vi "Generate Report.vi"(7 "Data_In":T1={"Input Data 1D"=[], "Channel Settings"={"Supply Voltage [Vdc]"=0.0, "Max Supply Current [Idc]"=0.0, "Settling Delay"=0.0, "Temp Criteria"=0.0, "Voltage Steps [Vrms]"=[0.0, 0.25, 0.5, 1.0, 1.95, 3.0, 3.9, 5.5], "User Notes"="", "Config Wave File Path"=path "C:/ASD Power Point Beta 32J/Waveforms/150HzSine5Second.wav", "Config Voltage [Vrms]"=0.0, "Channel Configuration List"={"Channel Configuration Cluster"={"Input"=enum."---", "Enable"=FALSE, "User Notes"="", "Voltage Range"=0.0, "Current Range"=2.5}, "Channel Configuration Cluster 2"={"Input"=enum."---", "Enable"=FALSE, "User Notes"="", "Voltage Range"=0.0, "Current Range"=2.5}, "Channel Configuration Cluster 3"={"Input"=enum."---", "Enable"=FALSE, "User Notes"="", "Voltage Range"=0.0, "Current Range"=2.5}, "Channel Configuration Cluster 4"={"Input"=enum."---", "Enable"=FALSE, "User Notes"="", "Voltage Range"=0.0, "Current Range"=2.5}, "Channel Configuration Cluster 5"={"Input"=enum."---", "Enable"=FALSE, "User Notes"="", "Voltage Range"=0.0, "Current Range"=2.5}, "Channel Configuration Cluster 6"={"Input"=enum."---", "Enable"=FALSE, "User Notes"="", "Voltage Range"=0.0, "Current Range"=2.5}, "Channel Configuration Cluster 7"={"Input"=enum."---", "Enable"=FALSE, "User Notes"="", "Voltage Range"=0.0, "Current Range"=2.5}, "Channel Configuration Cluster 8"={"Input"=enum."---", "Enable"=FALSE, "User Notes"="", "Voltage Range"=0.0, "Current Range"=2.5}, "Channel Configuration Cluster 9"={"Input"=enum."---", "Enable"=FALSE, "User Notes"="", "Voltage Range"=0.0, "Current Range"=2.5}, "Channel Configuration Cluster 10"={"Input"=enum."---", "Enable"=FALSE, "User Notes"="", "Voltage Range"=0.0, "Current Range"=2.5}, "Channel Configuration Cluster 11"={"Input"=enum."---", "Enable"=FALSE, "User Notes"="", "Voltage Range"=0.0, "Current Range"=2.5}, "Channel Configuration Cluster 12"={"Input"=enum."---", "Enable"=FALSE, "User Notes"="", "Voltage Range"=0.0, "Current Range"=2.5}, "Channel Configuration Cluster 13"={"Input"=enum."---", "Enable"=FALSE, "User Notes"="", "Voltage Range"=0.0, "Current Range"=2.5}, "Channel Configuration Cluster 14"={"Input"=enum."---", "Enable"=FALSE, "User Notes"="", "Voltage Range"=0.0, "Current Range"=2.5}, "Channel Configuration Cluster 15"={"Input"=enum."---", "Enable"=FALSE, "User Notes"="", "Voltage Range"=0.0, "Current Range"=2.5}, "Channel Configuration Cluster 16"={"Input"=enum."---", "Enable"=FALSE, "User Notes"="", "Voltage Range"=0.0, "Current Range"=2.5}, "Channel Configuration Cluster 17"={"Input"=enum."---", "Enable"=FALSE, "User Notes"="", "Voltage Range"=0.0, "Current Range"=2.5}}, "User Gains"={"Gain 1"=0.0, "Gain 2"=0.0, "Gain 3"=0.0, "Gain 4"=0.0, "Gain 5"=0.0, "Gain 6"=0.0}, "Gains"={"Gain 1"=0.0, "Gain 2"=0.0, "Gain 3"=0.0, "Gain 4"=0.0, "Gain 5"=0.0, "Gain 6"=0.0}, "Gain Array"={"Gain 1"=0.0, "Gain 2"=0.0, "Gain 3"=0.0, "Gain 4"=0.0, "Gain 5"=0.0, "Gain 6"=0.0, "Gain 7"=0.0, "Gain 8"=0.0, "Gain 9"=0.0, "Gain 10"=0.0, "Gain 11"=0.0, "Gain 12"=0.0, "Gain 13"=0.0, "Gain 14"=0.0, "Gain 15"=0.0, "Gain 16"=0.0, "Gain 17"=0.0}, "Wave File Path 1"=path "", "Wave File Path 2"=path "", "Wave File Path 3"=path "", "Wave File Path 4"=path "", "Range"=FALSE, "CF"=FALSE}, "Select Data"={"Vrms Data"=FALSE, "Vpkpk Data"=FALSE, "Irms Data"=FALSE, "Power Data"=FALSE, "Ipkpk Data"=FALSE, "Temp Data"=FALSE}, "Detailed Report ?"=FALSE, "Path Settings:"={"Template Path "=path "E:/L&T Projects/Bose ASD/Excel Template/ASD Template.xltx", "Report Path"=path "E:/L&T Projects/Bose ASD/excel Reports", "JPEG1 Path "=path "C:/Users/Public/Pictures/Sample Pictures/Hydrangeas.jpg", "JPEG2 Path"=path "C:/Users/Public/Pictures/Sample Pictures/Lighthouse.jpg"}, "Vrms_Sheet"=[], "Irms_Sheet"=[], "Power_Sheet"=[], "Vpk_Sheet"=[], "Ipk_Sheet"=[], "Vrms_Avg"=[], "Irms_Avg"=[], "Power_Avg"=[], "Vpk_Avg"=[], "Ipk_Avg"=[], "Report_Ref"=refnum, "User Name"="", "Temp_Sheet"=[]} {"Channel Settings"."Gain Array"."Gain 17" format="%.2f"; "Channel Settings"."Gain Array"."Gain 16" format="%.2f"; "Channel Settings"."Gain Array"."Gain 15" format="%.2f"; "Channel Settings"."Gain Array"."Gain 14" format="%.2f"; "Channel Settings"."Gain Array"."Gain 13" format="%.2f"; "Channel Settings"."Gain Array"."Gain 12" format="%.2f"; "Channel Settings"."Gain Array"."Gain 11" format="%.2f"; "Channel Settings"."Gain Array"."Gain 10" format="%.2f"; "Channel Settings"."Gain Array"."Gain 9" format="%.2f"; "Channel Settings"."Gain Array"."Gain 8" format="%.2f"; "Channel Settings"."Gain Array"."Gain 7" format="%.2f"; "Channel Settings"."Gain Array"."Gain 6" format="%.2f"; "Channel Settings"."Gain Array"."Gain 5" format="%.2f"; "Channel Settings"."Gain Array"."Gain 4" format="%.2f"; "Channel Settings"."Gain Array"."Gain 3" format="%.2f"; "Channel Settings"."Gain Array"."Gain 2" format="%.2f"; "Channel Settings"."Gain Array"."Gain 1" format="%.2f"; "Channel Settings"."Gains"."Gain 6" format="%.2f"; "Channel Settings"."Gains"."Gain 5" format="%.2f"; "Channel Settings"."Gains"."Gain 4" format="%.2f"; "Channel Settings"."Gains"."Gain 3" format="%.2f"; "Channel Settings"."Gains"."Gain 2" format="%.2f"; "Channel Settings"."Gains"."Gain 1" format="%.2f"; "Channel Settings"."User Gains"."Gain 6" format="%.2f"; "Channel Settings"."User Gains"."Gain 5" format="%.2f"; "Channel Settings"."User Gains"."Gain 4" format="%.2f"; "Channel Settings"."User Gains"."Gain 3" format="%.2f"; "Channel Settings"."User Gains"."Gain 2" format="%.2f"; "Channel Settings"."User Gains"."Gain 1" format="%.2f"; "Channel Settings"."Channel Configuration List"."Channel Configuration Cluster 17"."Current Range" items=["1 <500m>"=0.5, "2 <1>"=1.0, "5 <2.5>"=2.5, "10 <5>"=5.0, "20 <10>"=10.0, "50 <25>"=25.0]; "Channel Settings"."Channel Configuration List"."Channel Configuration Cluster 17"."Voltage Range" items=["1.5 <0.75>"=0.75, "3 <1.5>"=1.5, "6 <3>"=3.0, "10 <5>"=5.0, "15 <7.5>"=7.5, "30 <15>"=15.0, "60 <30>"=30.0, "100 <50>"=50.0, "150 <75>"=75.0, "300 <150>"=150.0, "600 <300>"=300.0, "1000 <500>"=500.0]; "Channel Settings"."Channel Configuration List"."Channel Configuration Cluster 16"."Current Range" items=["1 <500m>"=0.5, "2 <1>"=1.0, "5 <2.5>"=2.5, "10 <5>"=5.0, "20 <10>"=10.0, "50 <25>"=25.0]; "Channel Settings"."Channel Configuration List"."Channel Configuration Cluster 16"."Voltage Range" items=["1.5 <0.75>"=0.75, "3 <1.5>"=1.5, "6 <3>"=3.0, "10 <5>"=5.0, "15 <7.5>"=7.5, "30 <15>"=15.0, "60 <30>"=30.0, "100 <50>"=50.0, "150 <75>"=75.0, "300 <150>"=150.0, "600 <300>"=300.0, "1000 <500>"=500.0]; "Channel Settings"."Channel Configuration List"."Channel Configuration Cluster 15"."Current Range" items=["1 <500m>"=0.5, "2 <1>"=1.0, "5 <2.5>"=2.5, "10 <5>"=5.0, "20 <10>"=10.0, "50 <25>"=25.0]; "Channel Settings"."Channel Configuration List"."Channel Configuration Cluster 15"."Voltage Range" items=["1.5 <0.75>"=0.75, "3 <1.5>"=1.5, "6 <3>"=3.0, "10 <5>"=5.0, "15 <7.5>"=7.5, "30 <15>"=15.0, "60 <30>"=30.0, "100 <50>"=50.0, "150 <75>"=75.0, "300 <150>"=150.0, "600 <300>"=300.0, "1000 <500>"=500.0]; "Channel Settings"."Channel Configuration List"."Channel Configuration Cluster 14"."Current Range" items=["1 <500m>"=0.5, "2 <1>"=1.0, "5 <2.5>"=2.5, "10 <5>"=5.0, "20 <10>"=10.0, "50 <25>"=25.0]; "Channel Settings"."Channel Configuration List"."Channel Configuration Cluster 14"."Voltage Range" items=["1.5 <0.75>"=0.75, "3 <1.5>"=1.5, "6 <3>"=3.0, "10 <5>"=5.0, "15 <7.5>"=7.5, "30 <15>"=15.0, "60 <30>"=30.0, "100 <50>"=50.0, "150 <75>"=75.0, "300 <150>"=150.0, "600 <300>"=300.0, "1000 <500>"=500.0]; "Channel Settings"."Channel Configuration List"."Channel Configuration Cluster 13"."Current Range" items=["1 <500m>"=0.5, "2 <1>"=1.0, "5 <2.5>"=2.5, "10 <5>"=5.0, "20 <10>"=10.0, "50 <25>"=25.0]; "Channel Settings"."Channel Configuration List"."Channel Configuration Cluster 13"."Voltage Range" items=["1.5 <0.75>"=0.75, "3 <1.5>"=1.5, "6 <3>"=3.0, "10 <5>"=5.0, "15 <7.5>"=7.5, "30 <15>"=15.0, "60 <30>"=30.0, "100 <50>"=50.0, "150 <75>"=75.0, "300 <150>"=150.0, "600 <300>"=300.0, "1000 <500>"=500.0]; "Channel Settings"."Channel Configuration List"."Channel Configuration Cluster 12"."Current Range" items=["1 <500m>"=0.5, "2 <1>"=1.0, "5 <2.5>"=2.5, "10 <5>"=5.0, "20 <10>"=10.0, "50 <25>"=25.0]; "Channel Settings"."Channel Configuration List"."Channel Configuration Cluster 12"."Voltage Range" items=["1.5 <0.75>"=0.75, "3 <1.5>"=1.5, "6 <3>"=3.0, "10 <5>"=5.0, "15 <7.5>"=7.5, "30 <15>"=15.0, "60 <30>"=30.0, "100 <50>"=50.0, "150 <75>"=75.0, "300 <150>"=150.0, "600 <300>"=300.0, "1000 <500>"=500.0]; "Channel Settings"."Channel Configuration List"."Channel Configuration Cluster 11"."Current Range" items=["1 <500m>"=0.5, "2 <1>"=1.0, "5 <2.5>"=2.5, "10 <5>"=5.0, "20 <10>"=10.0, "50 <25>"=25.0]; "Channel Settings"."Channel Configuration List"."Channel Configuration Cluster 11"."Voltage Range" items=["1.5 <0.75>"=0.75, "3 <1.5>"=1.5, "6 <3>"=3.0, "10 <5>"=5.0, "15 <7.5>"=7.5, "30 <15>"=15.0, "60 <30>"=30.0, "100 <50>"=50.0, "150 <75>"=75.0, "300 <150>"=150.0, "600 <300>"=300.0, "1000 <500>"=500.0]; "Channel Settings"."Channel Configuration List"."Channel Configuration Cluster 10"."Current Range" items=["1 <500m>"=0.5, "2 <1>"=1.0, "5 <2.5>"=2.5, "10 <5>"=5.0, "20 <10>"=10.0, "50 <25>"=25.0]; "Channel Settings"."Channel Configuration List"."Channel Configuration Cluster 10"."Voltage Range" items=["1.5 <0.75>"=0.75, "3 <1.5>"=1.5, "6 <3>"=3.0, "10 <5>"=5.0, "15 <7.5>"=7.5, "30 <15>"=15.0, "60 <30>"=30.0, "100 <50>"=50.0, "150 <75>"=75.0, "300 <150>"=150.0, "600 <300>"=300.0, "1000 <500>"=500.0]; "Channel Settings"."Channel Configuration List"."Channel Configuration Cluster 9"."Voltage Range" items=["1.5 <0.75>"=0.75, "3 <1.5>"=1.5, "6 <3>"=3.0, "10 <5>"=5.0, "15 <7.5>"=7.5, "30 <15>"=15.0, "60 <30>"=30.0, "100 <50>"=50.0, "150 <75>"=75.0, "300 <150>"=150.0, "600 <300>"=300.0, "1000 <500>"=500.0]; "Channel Settings"."Channel Configuration List"."Channel Configuration Cluster 9"."Current Range" items=["10m <5m>"=0.005, "20m <10m>"=0.01, "50m <25m>"=0.025, "100m <50m>"=0.05, "200m <100m>"=0.1, "500m <250m>"=0.25, "1 <500m>"=0.5, "2 <1>"=1.0, "5 <2.5>"=2.5]; "Channel Settings"."Channel Configuration List"."Channel Configuration Cluster 8"."Voltage Range" items=["1.5 <0.75>"=0.75, "3 <1.5>"=1.5, "6 <3>"=3.0, "10 <5>"=5.0, "15 <7.5>"=7.5, "30 <15>"=15.0, "60 <30>"=30.0, "100 <50>"=50.0, "150 <75>"=75.0, "300 <150>"=150.0, "600 <300>"=300.0, "1000 <500>"=500.0]; "Channel Settings"."Channel Configuration List"."Channel Configuration Cluster 8"."Current Range" items=["10m <5m>"=0.005, "20m <10m>"=0.01, "50m <25m>"=0.025, "100m <50m>"=0.05, "200m <100m>"=0.1, "500m <250m>"=0.25, "1 <500m>"=0.5, "2 <1>"=1.0, "5 <2.5>"=2.5]; "Channel Settings"."Channel Configuration List"."Channel Configuration Cluster 7"."Voltage Range" items=["1.5 <0.75>"=0.75, "3 <1.5>"=1.5, "6 <3>"=3.0, "10 <5>"=5.0, "15 <7.5>"=7.5, "30 <15>"=15.0, "60 <30>"=30.0, "100 <50>"=50.0, "150 <75>"=75.0, "300 <150>"=150.0, "600 <300>"=300.0, "1000 <500>"=500.0]; "Channel Settings"."Channel Configuration List"."Channel Configuration Cluster 7"."Current Range" items=["10m <5m>"=0.005, "20m <10m>"=0.01, "50m <25m>"=0.025, "100m <50m>"=0.05, "200m <100m>"=0.1, "500m <250m>"=0.25, "1 <500m>"=0.5, "2 <1>"=1.0, "5 <2.5>"=2.5]; "Channel Settings"."Channel Configuration List"."Channel Configuration Cluster 6"."Voltage Range" items=["1.5 <0.75>"=0.75, "3 <1.5>"=1.5, "6 <3>"=3.0, "10 <5>"=5.0, "15 <7.5>"=7.5, "30 <15>"=15.0, "60 <30>"=30.0, "100 <50>"=50.0, "150 <75>"=75.0, "300 <150>"=150.0, "600 <300>"=300.0, "1000 <500>"=500.0]; "Channel Settings"."Channel Configuration List"."Channel Configuration Cluster 6"."Current Range" items=["10m <5m>"=0.005, "20m <10m>"=0.01, "50m <25m>"=0.025, "100m <50m>"=0.05, "200m <100m>"=0.1, "500m <250m>"=0.25, "1 <500m>"=0.5, "2 <1>"=1.0, "5 <2.5>"=2.5]; "Channel Settings"."Channel Configuration List"."Channel Configuration Cluster 5"."Voltage Range" items=["1.5 <0.75>"=0.75, "3 <1.5>"=1.5, "6 <3>"=3.0, "10 <5>"=5.0, "15 <7.5>"=7.5, "30 <15>"=15.0, "60 <30>"=30.0, "100 <50>"=50.0, "150 <75>"=75.0, "300 <150>"=150.0, "600 <300>"=300.0, "1000 <500>"=500.0]; "Channel Settings"."Channel Configuration List"."Channel Configuration Cluster 5"."Current Range" items=["10m <5m>"=0.005, "20m <10m>"=0.01, "50m <25m>"=0.025, "100m <50m>"=0.05, "200m <100m>"=0.1, "500m <250m>"=0.25, "1 <500m>"=0.5, "2 <1>"=1.0, "5 <2.5>"=2.5]; "Channel Settings"."Channel Configuration List"."Channel Configuration Cluster 4"."Voltage Range" items=["1.5 <0.75>"=0.75, "3 <1.5>"=1.5, "6 <3>"=3.0, "10 <5>"=5.0, "15 <7.5>"=7.5, "30 <15>"=15.0, "60 <30>"=30.0, "100 <50>"=50.0, "150 <75>"=75.0, "300 <150>"=150.0, "600 <300>"=300.0, "1000 <500>"=500.0]; "Channel Settings"."Channel Configuration List"."Channel Configuration Cluster 4"."Current Range" items=["10m <5m>"=0.005, "20m <10m>"=0.01, "50m <25m>"=0.025, "100m <50m>"=0.05, "200m <100m>"=0.1, "500m <250m>"=0.25, "1 <500m>"=0.5, "2 <1>"=1.0, "5 <2.5>"=2.5]; "Channel Settings"."Channel Configuration List"."Channel Configuration Cluster 3"."Voltage Range" items=["1.5 <0.75>"=0.75, "3 <1.5>"=1.5, "6 <3>"=3.0, "10 <5>"=5.0, "15 <7.5>"=7.5, "30 <15>"=15.0, "60 <30>"=30.0, "100 <50>"=50.0, "150 <75>"=75.0, "300 <150>"=150.0, "600 <300>"=300.0, "1000 <500>"=500.0]; "Channel Settings"."Channel Configuration List"."Channel Configuration Cluster 3"."Current Range" items=["10m <5m>"=0.005, "20m <10m>"=0.01, "50m <25m>"=0.025, "100m <50m>"=0.05, "200m <100m>"=0.1, "500m <250m>"=0.25, "1 <500m>"=0.5, "2 <1>"=1.0, "5 <2.5>"=2.5]; "Channel Settings"."Channel Configuration List"."Channel Configuration Cluster 2"."Voltage Range" items=["1.5 <0.75>"=0.75, "3 <1.5>"=1.5, "6 <3>"=3.0, "10 <5>"=5.0, "15 <7.5>"=7.5, "30 <15>"=15.0, "60 <30>"=30.0, "100 <50>"=50.0, "150 <75>"=75.0, "300 <150>"=150.0, "600 <300>"=300.0, "1000 <500>"=500.0]; "Channel Settings"."Channel Configuration List"."Channel Configuration Cluster 2"."Current Range" items=["10m <5m>"=0.005, "20m <10m>"=0.01, "50m <25m>"=0.025, "100m <50m>"=0.05, "200m <100m>"=0.1, "500m <250m>"=0.25, "1 <500m>"=0.5, "2 <1>"=1.0, "5 <2.5>"=2.5]; "Channel Settings"."Channel Configuration List"."Channel Configuration Cluster"."Voltage Range" items=["1.5 <0.75>"=0.75, "3 <1.5>"=1.5, "6 <3>"=3.0, "10 <5>"=5.0, "15 <7.5>"=7.5, "30 <15>"=15.0, "60 <30>"=30.0, "100 <50>"=50.0, "150 <75>"=75.0, "300 <150>"=150.0, "600 <300>"=300.0, "1000 <500>"=500.0]; "Channel Settings"."Channel Configuration List"."Channel Configuration Cluster"."Current Range" items=["10m <5m>"=0.005, "20m <10m>"=0.01, "50m <25m>"=0.025, "100m <50m>"=0.05, "200m <100m>"=0.1, "500m <250m>"=0.25, "1 <500m>"=0.5, "2 <1>"=1.0, "5 <2.5>"=2.5]; "Channel Settings"."Settling Delay" min=0.0 format="%<%H:%M:%S>t"; "Input Data 1D"."WT1800 Averages"."Vrms" format="%.3f"; "Input Data 1D"."WT1800 Averages"."Irms" format="%.3f"; "Input Data 1D"."WT1800 Averages"."Power" format="%.3f"; "Input Data 1D"."WT1800 Averages"."Vpkpk" format="%.3f"; "Input Data 1D"."WT1800 Averages"."Ipkpk" format="%.3f"; "Input Data 1D"."WT1800 Measurements"."Vrms" format="%.3f"; "Input Data 1D"."WT1800 Measurements"."Irms" format="%.3f"; "Input Data 1D"."WT1800 Measurements"."Power" format="%.3f"; "Input Data 1D"."WT1800 Measurements"."Vpkpk" format="%.3f"; "Input Data 1D"."WT1800 Measurements"."Ipkpk" format="%.3f"; "Input Data 1D"."DSA Averages"."Vrms" format="%.3f"; "Input Data 1D"."DSA Averages"."Vdc" format="%.3f"; "Input Data 1D"."DSA Averages"."Vpk+" format="%.3f"; "Input Data 1D"."DSA Averages"."Vpk-" format="%.3f"; "Input Data 1D"."DSA Averages"."Vpkpk" format="%.3f"; "Input Data 1D"."DSA Measurements"."Vrms" format="%.3f"; "Input Data 1D"."DSA Measurements"."Vdc" format="%.3f"; "Input Data 1D"."DSA Measurements"."Vpk+" format="%.3f"; "Input Data 1D"."DSA Measurements"."Vpk-" format="%.3f"; "Input Data 1D"."DSA Measurements"."Vpkpk" format="%.3f"}, 8 "error in":errorcluster) -> (0 "error out":errorcluster)   [LabVIEW 2021]
doc: "This VI generates the excel report"
uses:
  Datalog Controls/Data.ctl
  <vilib>/Utility/NIReport.llb/NI_report.lvclass
  Controls/Datalog Cluster Array.ctl
  Controls/Datalog Bundle Control.ctl
  Controls/WT1800 Functions.ctl
  Controls/WT1800 Measurements.ctl
  Controls/WT1800 Readings.ctl
  Controls/DSA Functions.ctl
  Controls/DSA Measurements.ctl
  Controls/DSA Readings.ctl
  Controls/Settings Control.ctl
  Controls/Channel Configuration List.ctl
  Controls/Channel Configuration Cluster.ctl
  Controls/Channel Configuration Cluster High Current.ctl
  Controls/Gain Averages.ctl
  Controls/Gain Array.ctl
  Datalog Controls/Select_Data.ctl
  <vilib>/Utility/miscctls.llb/LVPointTypeDef.ctl
  Datalog Controls/StateMachineStates.ctl
  <vilib>/Utility/NIReport.llb/Report Type.ctl
  <vilib>/Utility/NIReport.llb/Append Text Table to Report (wrap).vi
  <vilib>/Utility/NIReport.llb/Append Image to Report (path wrap).vi
  <vilib>/Utility/NIReport.llb/Excel/NI_Excel.lvclass
  <vilib>/Utility/NIReport.llb/NI_ReportGenerationCore.lvlib
panel:
  # "Please Wait. . ."
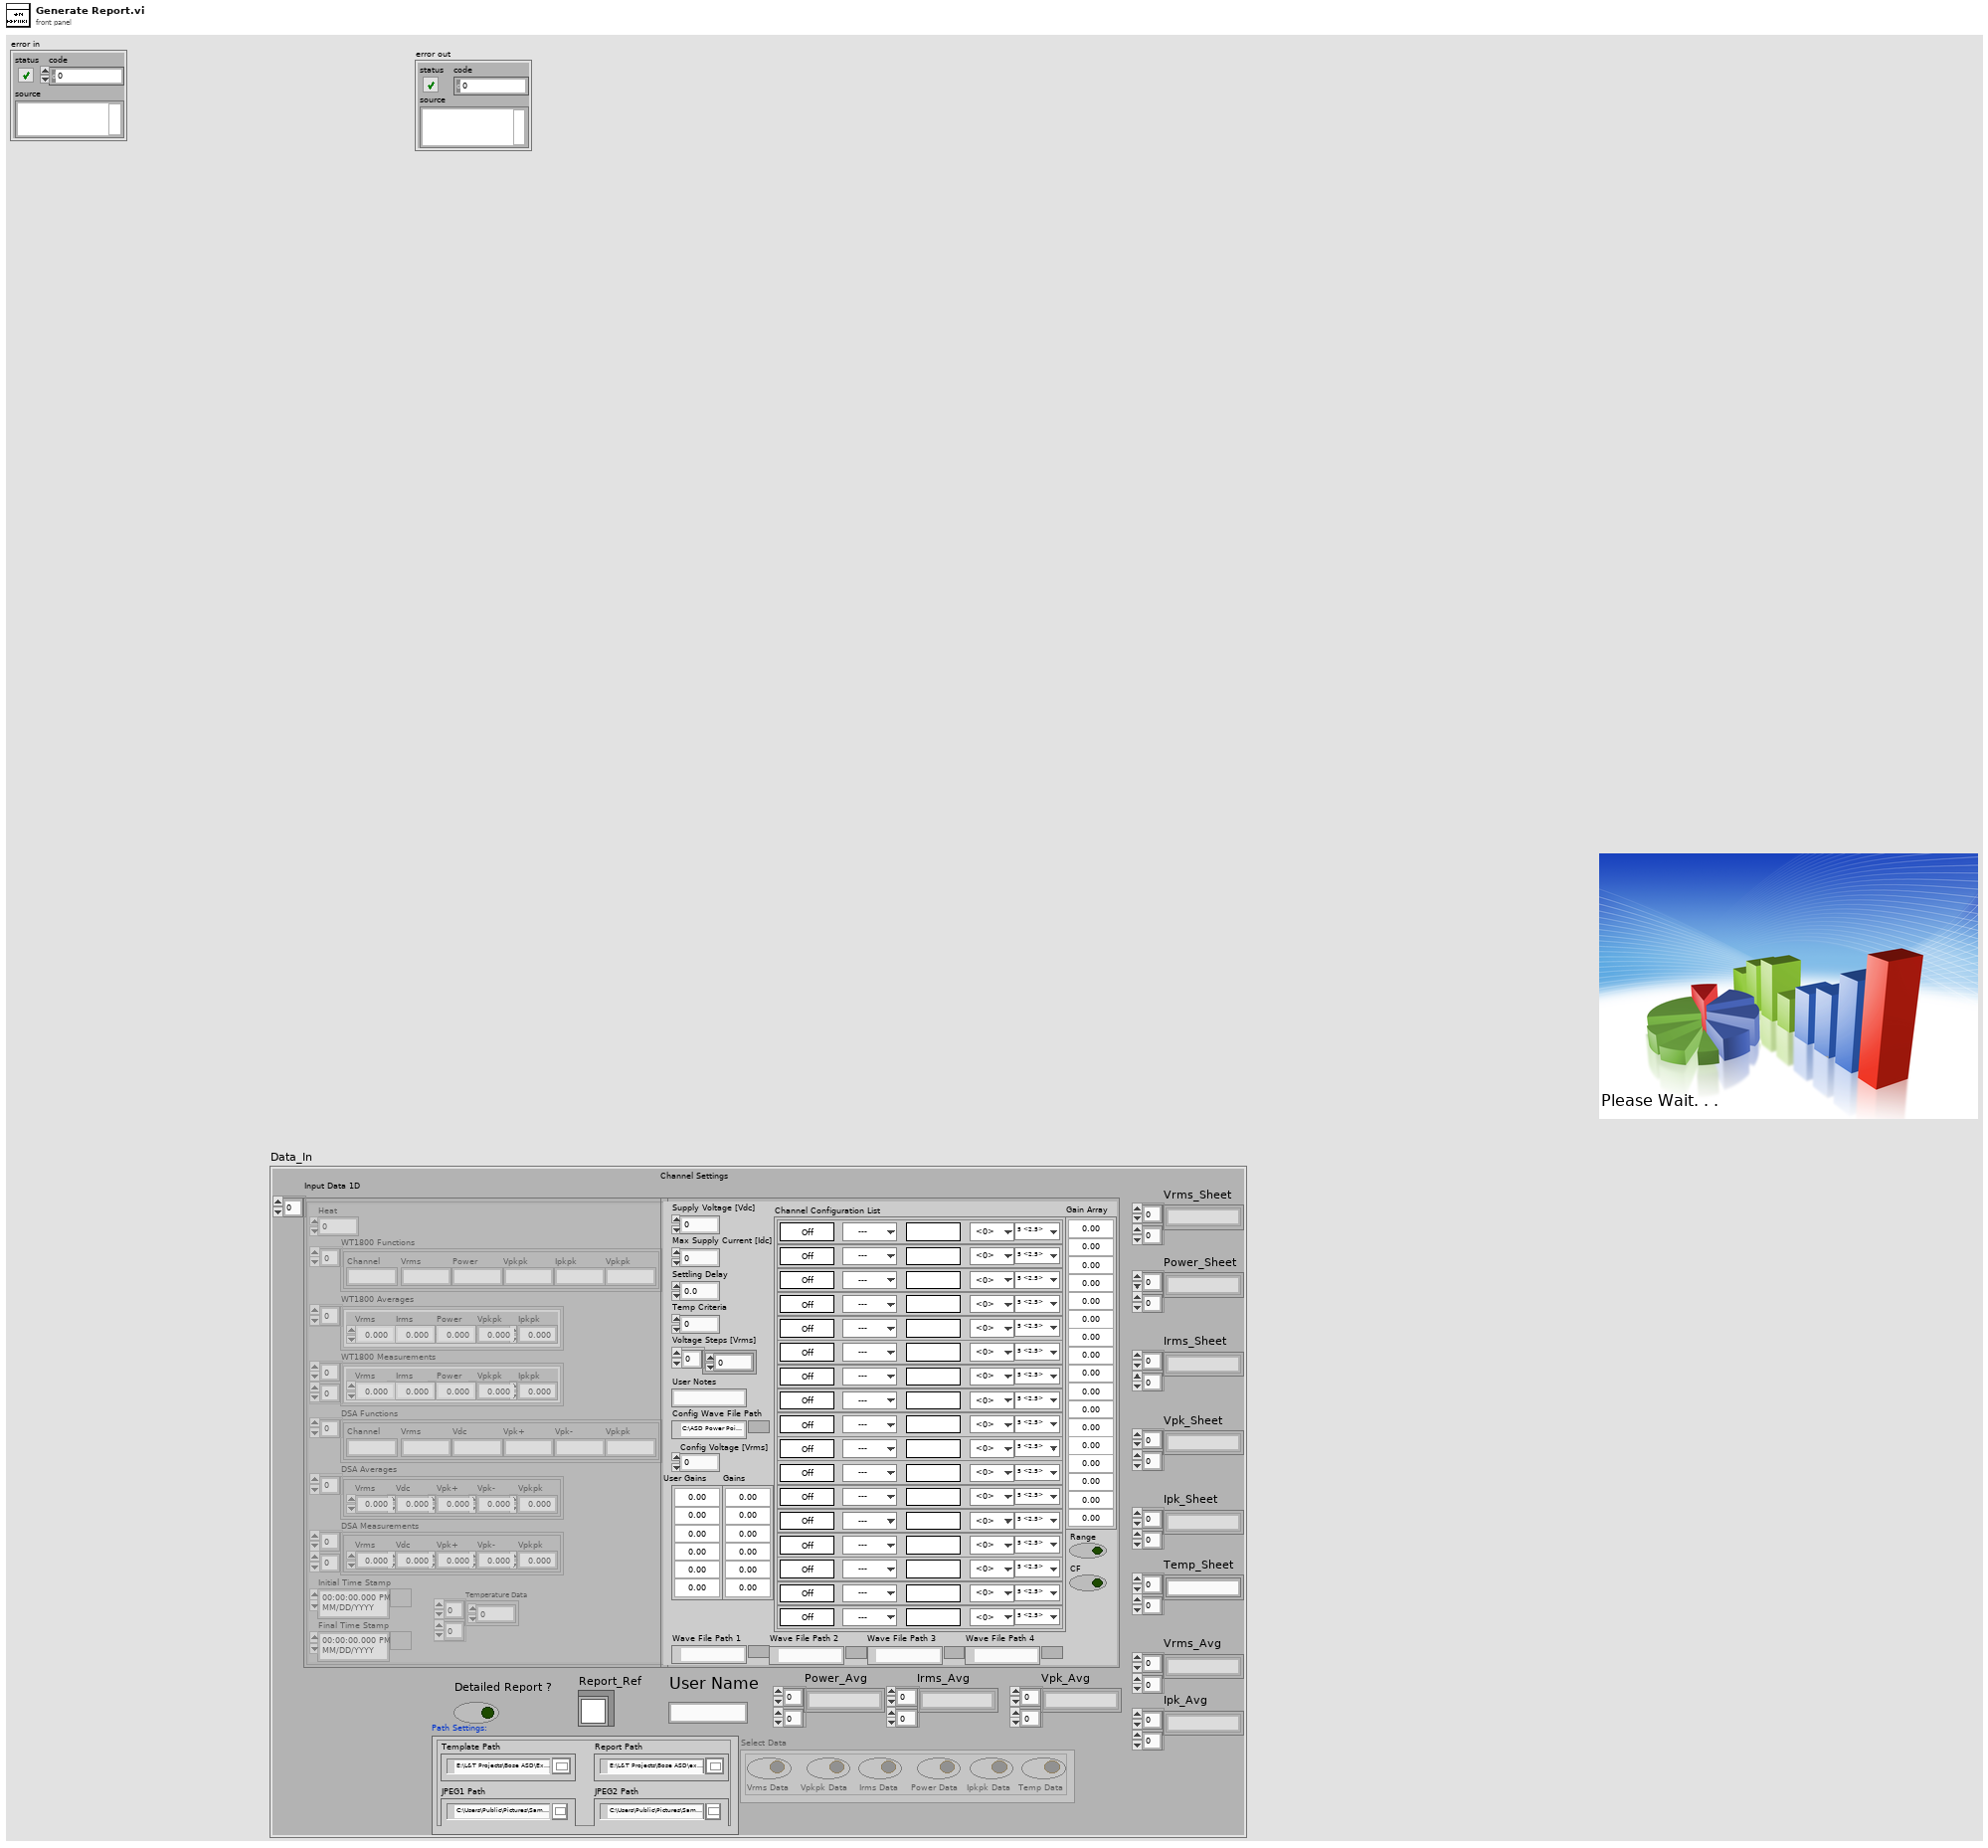
[diagram p1: front panel]
types:
  T1 = typedef "Data.ctl" = cluster{"Input Data 1D":T2, "Channel Settings":T10, "Select Data":T16, "Detailed Report ?":bool, "Path Settings:":cluster{"Template Path ":path, "Report Path":path, "JPEG1 Path ":path, "JPEG2 Path":path}, "Vrms_Sheet":string[][], "Irms_Sheet":string[][], "Power_Sheet":string[][], "Vpk_Sheet":string[][], "Ipk_Sheet":string[][], "Vrms_Avg":string[][], "Irms_Avg":string[][], "Power_Avg":string[][], "Vpk_Avg":string[][], "Ipk_Avg":string[][], "Report_Ref":refnum<class "NI_report.lvclass">, "User Name":string, "Temp_Sheet":string[][]}
  T2 = typedef "Datalog Cluster Array.ctl" = T3[]
  T3 = typedef "Datalog Bundle Control.ctl" = cluster{"Heat":dbl, "WT1800 Functions":T4, "WT1800 Averages":T5, "WT1800 Measurements":T6[][], "DSA Functions":T7, "DSA Averages":T8, "DSA Measurements":T9[][], "Initial Time Stamp":timestamp, "Final Time Stamp":timestamp, "Temperature Data":sgl[][]}
  T4 = typedef "WT1800 Functions.ctl" = cluster{"Channel":string, "Vrms":string, "Power":string, "Vpkpk":string, "Ipkpk":string, "Vpkpk":string}[]
  T5 = typedef "WT1800 Measurements.ctl" = T6[]
  T6 = typedef "WT1800 Readings.ctl" = cluster{"Vrms":sgl, "Irms":sgl, "Power":sgl, "Vpkpk":sgl, "Ipkpk":sgl}
  T7 = typedef "DSA Functions.ctl" = cluster{"Channel":string, "Vrms":string, "Vdc":string, "Vpk+":string, "Vpk-":string, "Vpkpk":string}[]
  T8 = typedef "DSA Measurements.ctl" = T9[]
  T9 = typedef "DSA Readings.ctl" = cluster{"Vrms":sgl, "Vdc":sgl, "Vpk+":sgl, "Vpk-":sgl, "Vpkpk":sgl}
  T10 = typedef "Settings Control.ctl" = cluster{"Supply Voltage [Vdc]":sgl, "Max Supply Current [Idc]":sgl, "Settling Delay":dbl, "Temp Criteria":sgl, "Voltage Steps [Vrms]":sgl[], "User Notes":string, "Config Wave File Path":path, "Config Voltage [Vrms]":sgl, "Channel Configuration List":T11, "User Gains":T14, "Gains":T14, "Gain Array":T15, "Wave File Path 1":path, "Wave File Path 2":path, "Wave File Path 3":path, "Wave File Path 4":path, "Range":bool, "CF":bool}
  T11 = typedef "Channel Configuration List.ctl" = cluster{"Channel Configuration Cluster":T12, "Channel Configuration Cluster 2":T12, "Channel Configuration Cluster 3":T12, "Channel Configuration Cluster 4":T12, "Channel Configuration Cluster 5":T12, "Channel Configuration Cluster 6":T12, "Channel Configuration Cluster 7":T12, "Channel Configuration Cluster 8":T12, "Channel Configuration Cluster 9":T12, "Channel Configuration Cluster 10":T13, "Channel Configuration Cluster 11":T13, "Channel Configuration Cluster 12":T13, "Channel Configuration Cluster 13":T13, "Channel Configuration Cluster 14":T13, "Channel Configuration Cluster 15":T13, "Channel Configuration Cluster 16":T13, "Channel Configuration Cluster 17":T13}
  T12 = typedef "Channel Configuration Cluster.ctl" = cluster{"Input":enum16{"---", "1", "1 AVG", "2", "2 AVG", "3", "3 AVG", "4", "4 AVG"}, "Enable":bool, "User Notes":string, "Voltage Range":dbl, "Current Range":dbl}
  T13 = typedef "Channel Configuration Cluster High Current.ctl" = cluster{"Input":enum16{"---", "1", "1 AVG", "2", "2 AVG", "3", "3 AVG", "4", "4 AVG"}, "Enable":bool, "User Notes":string, "Voltage Range":dbl, "Current Range":dbl}
  T14 = typedef "Gain Averages.ctl" = cluster{"Gain 1":dbl, "Gain 2":dbl, "Gain 3":dbl, "Gain 4":dbl, "Gain 5":dbl, "Gain 6":dbl}
  T15 = typedef "Gain Array.ctl" = cluster{"Gain 1":dbl, "Gain 2":dbl, "Gain 3":dbl, "Gain 4":dbl, "Gain 5":dbl, "Gain 6":dbl, "Gain 7":dbl, "Gain 8":dbl, "Gain 9":dbl, "Gain 10":dbl, "Gain 11":dbl, "Gain 12":dbl, "Gain 13":dbl, "Gain 14":dbl, "Gain 15":dbl, "Gain 16":dbl, "Gain 17":dbl}
  T16 = typedef "Select_Data.ctl" = cluster{"Vrms Data":bool, "Vpkpk Data":bool, "Irms Data":bool, "Power Data":bool, "Ipkpk Data":bool, "Temp Data":bool}
  T17 = typedef "StateMachineStates.ctl" = enum16{"Initialize", "Get Data", "Write Setup", "Write Vrms", "Write Irms", "Write Power", "Write Vpk", "Write Ipk", "Write Temp", "Append Images", "Write Summary", "Save", "Error", "Exit"}
  T18 = typedef "LVPointTypeDef.ctl" = cluster{"Horizontal":i16, "Vertical":i16}
  T19 = typedef "NI_ReportGenerationCore.lvlib/Report Type.ctl" = enum16{"HTML", "Word", "Excel"}
  T20 = enum16{"maximized", "minimized", "normal", "no change"}
  T21 = cluster{"position (excel)":cluster{"row":i32, "column":i32}, "name (excel)":string, "bookmark (word)":string}[]
  T22 = cluster{"position (excel)":cluster{"row":i32, "column":i32}, "name (excel)":string, "bookmark (word)":string}
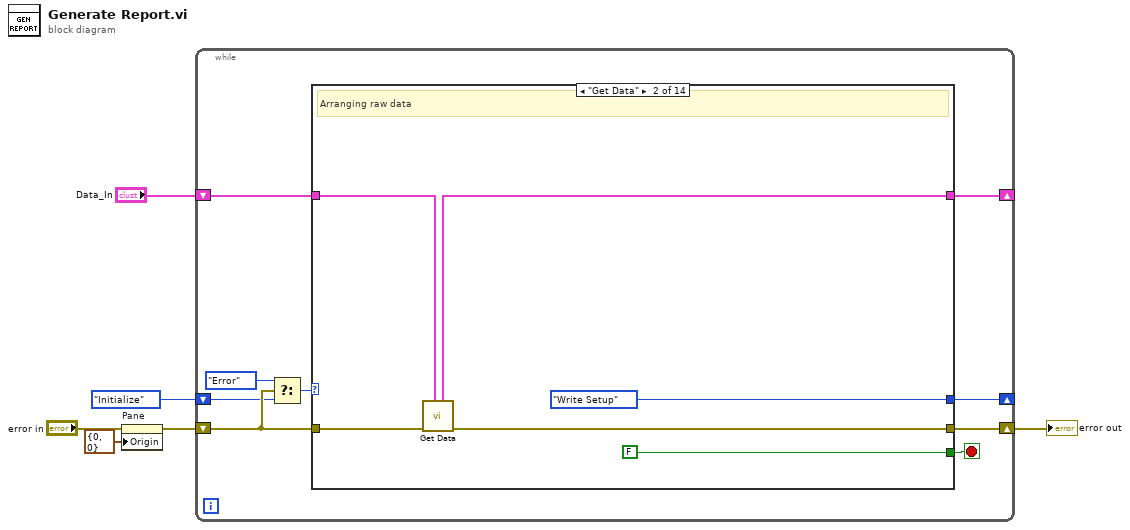
[diagram p0: block diagram]
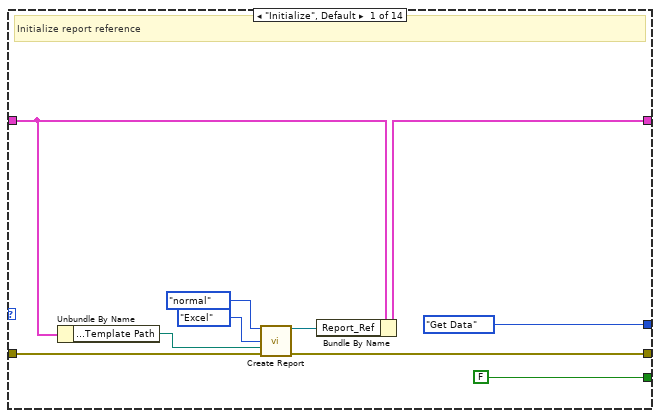
[diagram p2: hidden frame]
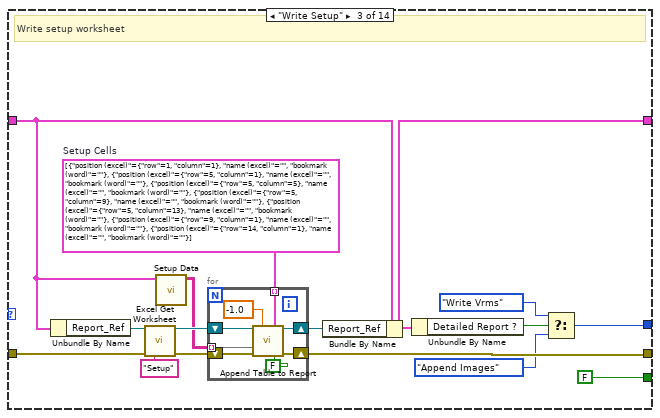
[diagram p3: hidden frame]
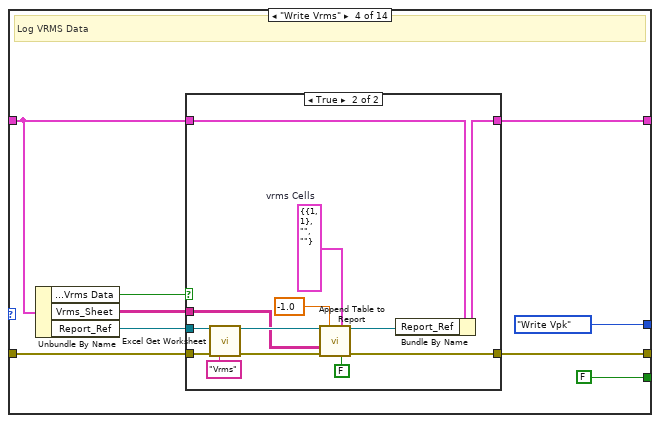
[diagram p4: hidden frame]
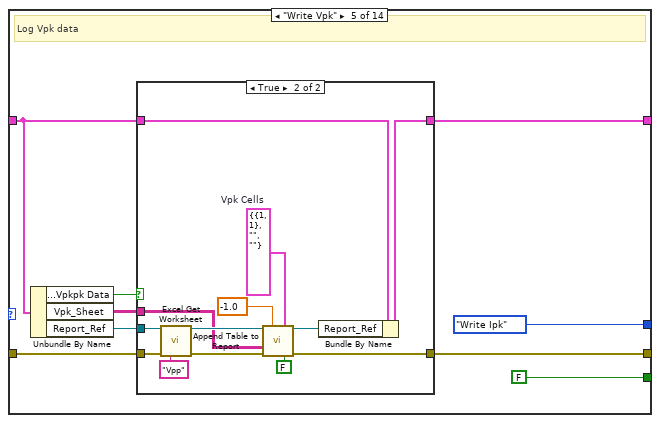
[diagram p6: hidden frame]
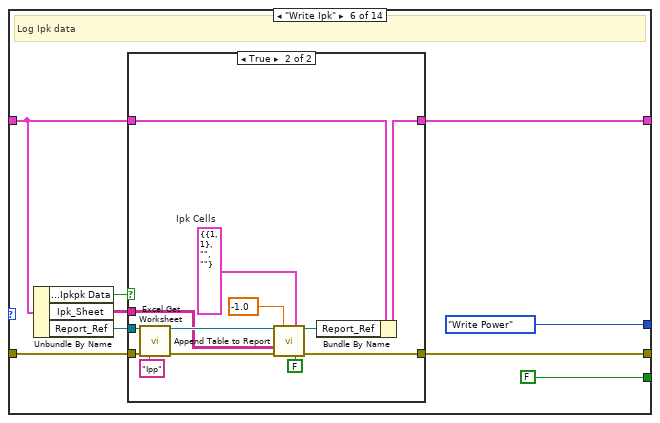
[diagram p8: hidden frame]
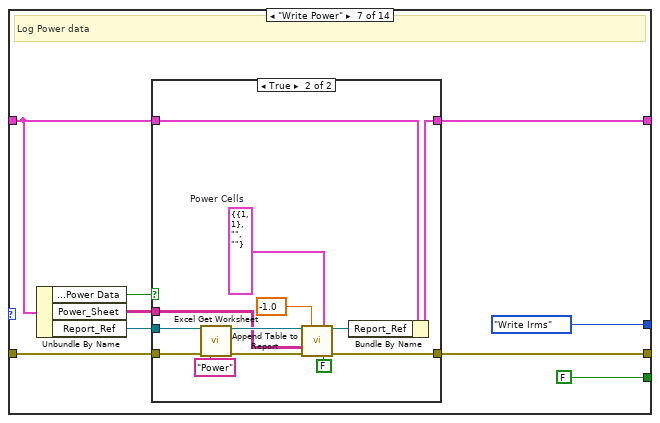
[diagram p10: hidden frame]
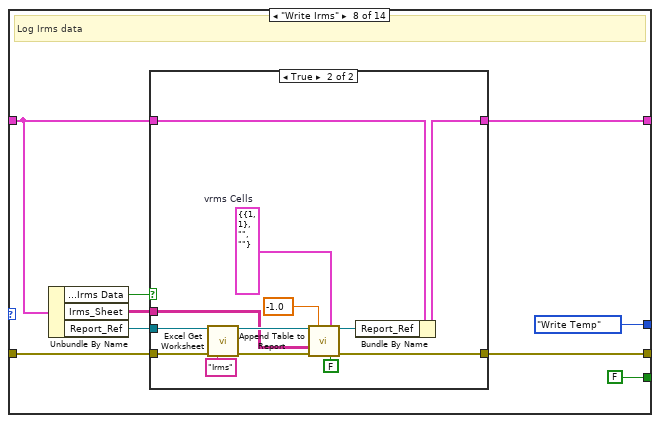
[diagram p12: hidden frame]
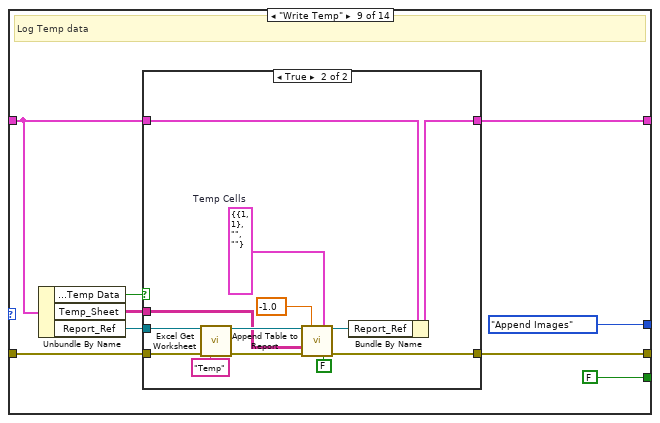
[diagram p14: hidden frame]
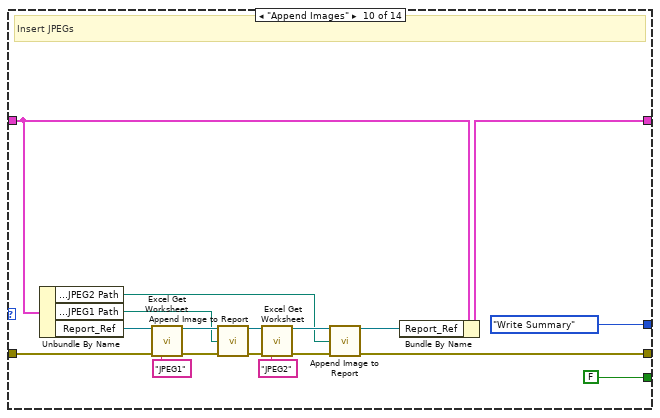
[diagram p16: hidden frame]
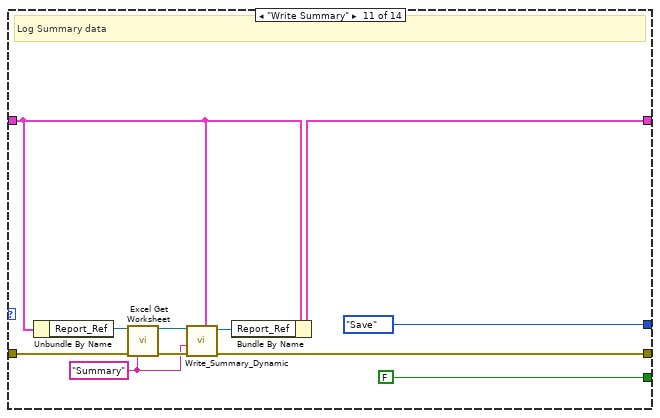
[diagram p17: hidden frame]
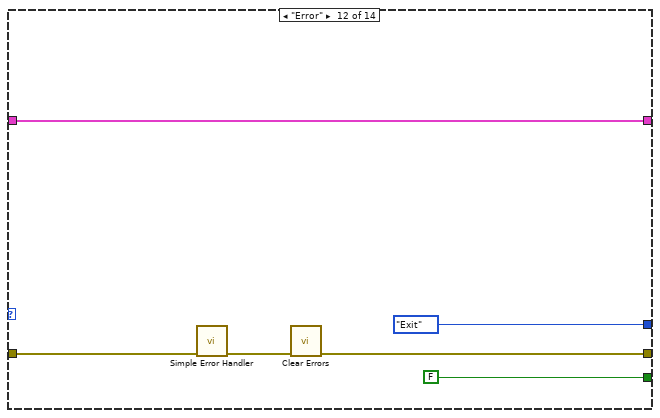
[diagram p18: hidden frame]
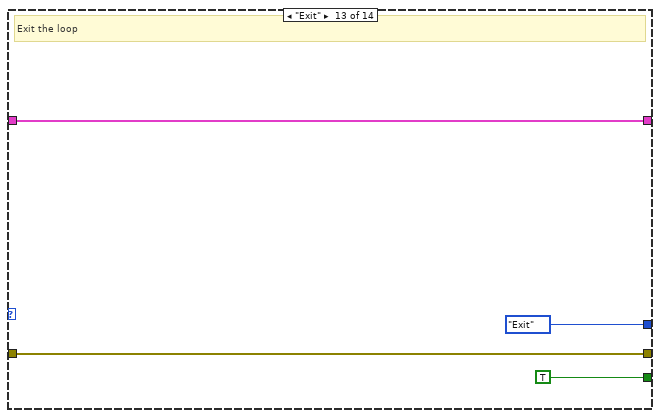
[diagram p19: hidden frame]
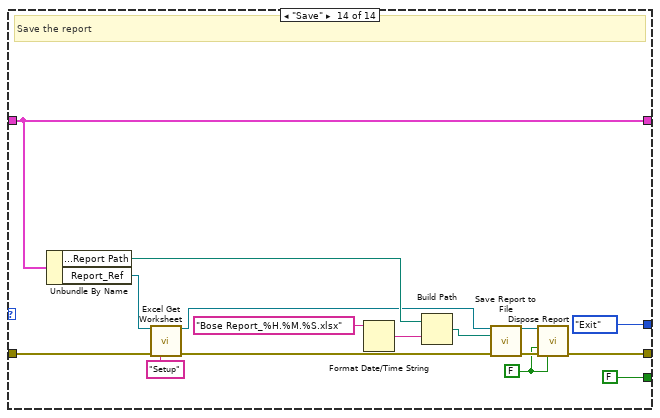
[diagram p20: hidden frame]
diagram:
  n1 = property on="Pane" class="Pane"(error in="error in", "Origin"=T18 {"Horizontal"=0, "Vertical"=0}) -> (error out=w3:errorcluster)  [unwired: 1 in, 1 out]
  n2 = while {
    shift-right: [w8] -> _
    shift-left: StateMachineStates."Initialize" ("t") -> [w10]
    shift-right: [w15] -> w6
    shift-left: w3 -> [w12]
    shift-right: [w13] -> _
    shift-left: "Data_In" -> [w14]
    stop <- w7 stop-if-true
    n3 = Select(t=StateMachineStates."Error", s=w12, f=w10) -> (s? t:f=w9:T17)
    n4 = case shown="\"Get Data\"" w9 {
      tunnel: w12 -> [w24 w30 w44 w64 w87 w112 w136 w160 w184 w216 w226 w234 w238 w242]
      tunnel: [w23 w29 w43 w63 w88 w111 w135 w159 w183 w206 w225 w232 w238 w252] -> w15
      tunnel: w14 -> [w19 w31 w34 w60 w84 w105 w132 w156 w180 w212 w222 w231 w235 w248]
      tunnel: [w21 w26 w40 w59 w83 w104 w131 w155 w179 w211 w221 w231 w235 w248] -> w13
      tunnel: [StateMachineStates."Get Data" ("t") StateMachineStates."Write Setup" ("t") w36 StateMachineStates."Write Vpk" ("t") StateMachineStates."Write Ipk" ("t") StateMachineStates."Write Power" ("t") StateMachineStates."Write Irms" ("t") StateMachineStates."Write Temp" ("t") StateMachineStates."Append Images" ("t") StateMachineStates."Write Summary" ("t") StateMachineStates."Save" ("t") StateMachineStates."Exit" ("t") StateMachineStates."Exit" ("t") StateMachineStates."Exit" ("t")] -> w8
      tunnel: [FALSE FALSE FALSE FALSE FALSE FALSE FALSE FALSE FALSE FALSE FALSE FALSE TRUE FALSE] -> w7
      frame "Initialize", Default {
        # "Initialize report reference"
        n5 = Unbundle By Name(w19) -> ("Path Settings:.Template Path"=w25:path)
        n6 = call <vilib>:"Create Report.vi"("window state (normal)"=T20."normal", "report type"=Report_Type."Excel", "template (empty)"=w25, "error in (no error)"=w24) -> ("report out"=w20:refnum<class "NI_report.lvclass">, "error out"=w23:errorcluster)  [unwired: 10 in]
        n7 = Bundle By Name(cluster=w19, "Report_Ref"=w20) -> (w21:T1)
      }
      frame "Get Data" {
        # "Arranging raw data"
        n8 = call "Get Data.vi"(7:w31, "error in"=w30) -> ("error out"=w29:errorcluster, "output cluster"=w26:T1)  [unwired: 8 in]
      }
      frame "Write Setup" {
        w32 = T21 [{"position (excel)"={"row"=1, "column"=1}, "name (excel)"="", "bookmark (word)"=""}, {"position (excel)"={"row"=5, "column"=1}, "name (excel)"="", "bookmark (word)"=""}, {"position (excel)"={"row"=5, "column"=5}, "name (excel)"="", "bookmark (word)"=""}, {"position (excel)"={"row"=5, "column"=9}, "name (excel)"="", "bookmark (word)"=""}, {"position (excel)"={"row"=5, "column"=13}, "name (excel)"="", "bookmark (word)"=""}, {"position (excel)"={"row"=9, "column"=1}, "name (excel)"="", "bookmark (word)"=""}, {"position (excel)"={"row"=14, "column"=1}, "name (excel)"="", "bookmark (word)"=""}]  # Setup Cells
        # "Write setup worksheet"
        n9 = Unbundle By Name(w34) -> ("Report_Ref"=w42:refnum<class "NI_report.lvclass">)
        n10 = call <vilib>:"Excel Get Worksheet.vi"("report in"=w42, "error in (no error)"=w44, "name (\"\")"="Setup" ("name (\"\")")) -> ("report out"=w46:refnum<class "NI_report.lvclass">, "error out"=w47:errorcluster)  [unwired: 11 in]
        n11 = call "Setup Data.vi"(11:w34) -> ("Set up data"=w33:string[][][])  [unwired: 10 in]
        n12 = for {
          tunnel: w33 -> [w51] mode=indexing
          tunnel: w32 -> [w48] mode=indexing
          shift-right: [w53] -> w43
          shift-left: w47 -> [w55]
          shift-right: [w52] -> w41
          shift-left: w46 -> [w54]
          n13 = call-poly <vilib>:"Append Table to Report.vi"("report in"=w54, "column width (1)"=-1.0, "MS Office parameters"=w48, "text data"=w51, "error in (no error)"=w55, "show grid lines (YES)"=FALSE) -> ("report out"=w52:refnum<class "NI_report.lvclass">, "error out"=w53:errorcluster)  [unwired: 6 in, 2 out]
        }
        n14 = Bundle By Name(cluster=w34, "Report_Ref"=w41) -> (w40:T1)
        n15 = Unbundle By Name(w40) -> ("Detailed Report ?"=w39:bool)
        n16 = Select(t=StateMachineStates."Write Vrms", s=w39, f=StateMachineStates."Append Images" ("t")) -> (s? t:f=w36:T17)
      }
      frame "Write Vrms" {
        # "Log VRMS Data"
        n17 = Unbundle By Name(w60) -> ("Select Data.Vrms Data"=w56:bool, "Vrms_Sheet"=w62:string[][], "Report_Ref"=w61:refnum<class "NI_report.lvclass">)
        n18 = case shown="True" w56 {
          tunnel: w64 -> [w65 w73]
          tunnel: [w65 w72] -> w63
          tunnel: w62 -> [_ w71]
          tunnel: w61 -> [_ w70]
          tunnel: w60 -> [w66 w68]
          tunnel: [w66 w67] -> w59
          frame False {
          }
          frame True {
            w76 = T22 {"position (excel)"={"row"=1, "column"=1}, "name (excel)"="", "bookmark (word)"=""}  # vrms Cells
            n19 = call <vilib>:"Excel Get Worksheet.vi"("report in"=w70, "error in (no error)"=w73, "name (\"\")"="Vrms" ("name (\"\")")) -> ("report out"=w78:refnum<class "NI_report.lvclass">, "error out"=w79:errorcluster)  [unwired: 11 in]
            n20 = call-poly <vilib>:"Append Table to Report.vi"("report in"=w78, "column width (1)"=-1.0, "MS Office parameters"=w76, "text data"=w71, "error in (no error)"=w79, "show grid lines (YES)"=FALSE) -> ("report out"=w69:refnum<class "NI_report.lvclass">, "error out"=w72:errorcluster)  [unwired: 6 in, 2 out]
            n21 = Bundle By Name(cluster=w68, "Report_Ref"=w69) -> (w67:T1)
          }
        }
      }
      frame "Write Vpk" {
        # "Log Vpk data"
        n22 = Unbundle By Name(w84) -> ("Select Data.Vpkpk Data"=w80:bool, "Vpk_Sheet"=w86:string[][], "Report_Ref"=w85:refnum<class "NI_report.lvclass">)
        n23 = case shown="True" w80 {
          tunnel: [w89 w97] -> w88
          tunnel: w87 -> [w89 w96]
          tunnel: w86 -> [_ w95]
          tunnel: w85 -> [_ w94]
          tunnel: w84 -> [w90 w92]
          tunnel: [w90 w91] -> w83
          frame False {
          }
          frame True {
            w100 = T22 {"position (excel)"={"row"=1, "column"=1}, "name (excel)"="", "bookmark (word)"=""}  # Vpk Cells
            n24 = call <vilib>:"Excel Get Worksheet.vi"("report in"=w94, "error in (no error)"=w96, "name (\"\")"="Vpp" ("name (\"\")")) -> ("report out"=w102:refnum<class "NI_report.lvclass">, "error out"=w103:errorcluster)  [unwired: 11 in]
            n25 = call-poly <vilib>:"Append Table to Report.vi"("report in"=w102, "column width (1)"=-1.0, "MS Office parameters"=w100, "text data"=w95, "error in (no error)"=w103, "show grid lines (YES)"=FALSE) -> ("report out"=w93:refnum<class "NI_report.lvclass">, "error out"=w97:errorcluster)  [unwired: 6 in, 2 out]
            n26 = Bundle By Name(cluster=w92, "Report_Ref"=w93) -> (w91:T1)
          }
        }
      }
      frame "Write Ipk" {
        # "Log Ipk data"
        n27 = Unbundle By Name(w105) -> ("Select Data.Ipkpk Data"=w106:bool, "Ipk_Sheet"=w109:string[][], "Report_Ref"=w110:refnum<class "NI_report.lvclass">)
        n28 = case shown="True" w106 {
          tunnel: w112 -> [w114 w121]
          tunnel: [w114 w120] -> w111
          tunnel: w110 -> [_ w119]
          tunnel: w109 -> [_ w118]
          tunnel: w105 -> [w113 w117]
          tunnel: [w113 w115] -> w104
          frame False {
          }
          frame True {
            w124 = T22 {"position (excel)"={"row"=1, "column"=1}, "name (excel)"="", "bookmark (word)"=""}  # Ipk Cells
            n29 = call <vilib>:"Excel Get Worksheet.vi"("report in"=w119, "error in (no error)"=w121, "name (\"\")"="Ipp" ("name (\"\")")) -> ("report out"=w126:refnum<class "NI_report.lvclass">, "error out"=w127:errorcluster)  [unwired: 11 in]
            n30 = call-poly <vilib>:"Append Table to Report.vi"("report in"=w126, "column width (1)"=-1.0, "MS Office parameters"=w124, "text data"=w118, "error in (no error)"=w127, "show grid lines (YES)"=FALSE) -> ("report out"=w116:refnum<class "NI_report.lvclass">, "error out"=w120:errorcluster)  [unwired: 6 in, 2 out]
            n31 = Bundle By Name(cluster=w117, "Report_Ref"=w116) -> (w115:T1)
          }
        }
      }
      frame "Write Power" {
        # "Log Power data"
        n32 = Unbundle By Name(w132) -> ("Select Data.Power Data"=w128:bool, "Power_Sheet"=w134:string[][], "Report_Ref"=w133:refnum<class "NI_report.lvclass">)
        n33 = case shown="True" w128 {
          tunnel: w136 -> [w138 w145]
          tunnel: [w138 w144] -> w135
          tunnel: w134 -> [_ w143]
          tunnel: w133 -> [_ w142]
          tunnel: w132 -> [w137 w141]
          tunnel: [w137 w139] -> w131
          frame False {
          }
          frame True {
            w148 = T22 {"position (excel)"={"row"=1, "column"=1}, "name (excel)"="", "bookmark (word)"=""}  # Power Cells
            n34 = call <vilib>:"Excel Get Worksheet.vi"("report in"=w142, "error in (no error)"=w145, "name (\"\")"="Power" ("name (\"\")")) -> ("report out"=w150:refnum<class "NI_report.lvclass">, "error out"=w151:errorcluster)  [unwired: 11 in]
            n35 = call-poly <vilib>:"Append Table to Report.vi"("report in"=w150, "column width (1)"=-1.0, "MS Office parameters"=w148, "text data"=w143, "error in (no error)"=w151, "show grid lines (YES)"=FALSE) -> ("report out"=w140:refnum<class "NI_report.lvclass">, "error out"=w144:errorcluster)  [unwired: 6 in, 2 out]
            n36 = Bundle By Name(cluster=w141, "Report_Ref"=w140) -> (w139:T1)
          }
        }
      }
      frame "Write Irms" {
        # "Log Irms data"
        n37 = Unbundle By Name(w156) -> ("Select Data.Irms Data"=w152:bool, "Irms_Sheet"=w158:string[][], "Report_Ref"=w157:refnum<class "NI_report.lvclass">)
        n38 = case shown="True" w152 {
          tunnel: w160 -> [w161 w169]
          tunnel: [w161 w168] -> w159
          tunnel: w158 -> [_ w167]
          tunnel: w157 -> [_ w166]
          tunnel: w156 -> [w162 w165]
          tunnel: [w162 w163] -> w155
          frame False {
          }
          frame True {
            w172 = T22 {"position (excel)"={"row"=1, "column"=1}, "name (excel)"="", "bookmark (word)"=""}  # vrms Cells
            n39 = call <vilib>:"Excel Get Worksheet.vi"("report in"=w166, "error in (no error)"=w169, "name (\"\")"="Irms" ("name (\"\")")) -> ("report out"=w174:refnum<class "NI_report.lvclass">, "error out"=w175:errorcluster)  [unwired: 11 in]
            n40 = call-poly <vilib>:"Append Table to Report.vi"("report in"=w174, "column width (1)"=-1.0, "MS Office parameters"=w172, "text data"=w167, "error in (no error)"=w175, "show grid lines (YES)"=FALSE) -> ("report out"=w164:refnum<class "NI_report.lvclass">, "error out"=w168:errorcluster)  [unwired: 6 in, 2 out]
            n41 = Bundle By Name(cluster=w165, "Report_Ref"=w164) -> (w163:T1)
          }
        }
      }
      frame "Write Temp" {
        # "Log Temp data"
        n42 = Unbundle By Name(w180) -> ("Select Data.Temp Data"=w176:bool, "Temp_Sheet"=w182:string[][], "Report_Ref"=w181:refnum<class "NI_report.lvclass">)
        n43 = case shown="True" w176 {
          tunnel: w184 -> [w185 w193]
          tunnel: [w185 w192] -> w183
          tunnel: w182 -> [_ w191]
          tunnel: w181 -> [_ w190]
          tunnel: w180 -> [w186 w189]
          tunnel: [w186 w187] -> w179
          frame False {
          }
          frame True {
            w196 = T22 {"position (excel)"={"row"=1, "column"=1}, "name (excel)"="", "bookmark (word)"=""}  # Temp Cells
            n44 = call <vilib>:"Excel Get Worksheet.vi"("report in"=w190, "error in (no error)"=w193, "name (\"\")"="Temp" ("name (\"\")")) -> ("report out"=w198:refnum<class "NI_report.lvclass">, "error out"=w199:errorcluster)  [unwired: 11 in]
            n45 = call-poly <vilib>:"Append Table to Report.vi"("report in"=w198, "column width (1)"=-1.0, "MS Office parameters"=w196, "text data"=w191, "error in (no error)"=w199, "show grid lines (YES)"=FALSE) -> ("report out"=w188:refnum<class "NI_report.lvclass">, "error out"=w192:errorcluster)  [unwired: 6 in, 2 out]
            n46 = Bundle By Name(cluster=w189, "Report_Ref"=w188) -> (w187:T1)
          }
        }
      }
      frame "Append Images" {
        # "Insert JPEGs"
        n47 = Unbundle By Name(w212) -> ("Path Settings:.JPEG2 Path"=w202:path, "Path Settings:.JPEG1 Path"=w203:path, "Report_Ref"=w213:refnum<class "NI_report.lvclass">)
        n48 = call <vilib>:"Excel Get Worksheet.vi"("report in"=w213, "error in (no error)"=w216, "name (\"\")"="JPEG1" ("name (\"\")")) -> ("report out"=w214:refnum<class "NI_report.lvclass">, "error out"=w215:errorcluster)  [unwired: 11 in]
        n49 = call-poly <vilib>:"Append Image to Report.vi"("report in"=w214, "path or URL of image"=w203, "error in (no error)"=w215) -> ("report out"=w205:refnum<class "NI_report.lvclass">, "error out"=w207:errorcluster)  [unwired: 9 in, 2 out]
        n50 = call <vilib>:"Excel Get Worksheet.vi"("report in"=w205, "error in (no error)"=w207, "name (\"\")"="JPEG2" ("name (\"\")")) -> ("report out"=w210:refnum<class "NI_report.lvclass">, "error out"=w209:errorcluster)  [unwired: 11 in]
        n51 = call-poly <vilib>:"Append Image to Report.vi"("report in"=w210, "path or URL of image"=w202, "error in (no error)"=w209) -> ("report out"=w204:refnum<class "NI_report.lvclass">, "error out"=w206:errorcluster)  [unwired: 9 in, 2 out]
        n52 = Bundle By Name(cluster=w212, "Report_Ref"=w204) -> (w211:T1)
      }
      frame "Write Summary" {
        w218 = "Summary" ("name (\"\")")
        # "Log Summary data"
        n53 = Unbundle By Name(w222) -> ("Report_Ref"=w224:refnum<class "NI_report.lvclass">)
        n54 = call <vilib>:"Excel Get Worksheet.vi"("report in"=w224, "error in (no error)"=w226, "name (\"\")"=w218) -> ("report out"=w227:refnum<class "NI_report.lvclass">, "error out"=w228:errorcluster)  [unwired: 11 in]
        n55 = call "Write_Summary_Dynamic.vi"("error in"=w228, "Sheet Name"=w218, "Data_In"=w222, "NI_report in"=w227) -> ("error out"=w225:errorcluster, "NI_report out"=w223:refnum<class "NI_report.lvclass">)  [unwired: 6 in]
        n56 = Bundle By Name(cluster=w222, "Report_Ref"=w223) -> (w221:T1)
      }
      frame "Error" {
        n57 = call <vilib>:"Simple Error Handler.vi"("error in (no error)"=w234) -> ("error out"=w233:errorcluster)  [unwired: 4 in, 4 out]
        n58 = call <vilib>:"Clear Errors.vi"("error in (no error)"=w233) -> ("error out"=w232:errorcluster)  [unwired: 5 in, 1 out]
      }
      frame "Exit" {
        # "Exit the loop"
      }
      frame "Save" {
        w247 = FALSE ("close report? (T)")
        # "Save the report"
        n59 = Unbundle By Name(w248) -> ("Path Settings:.Report Path"=w246:path, "Report_Ref"=w239:refnum<class "NI_report.lvclass">)
        n60 = call <vilib>:"Excel Get Worksheet.vi"("report in"=w239, "error in (no error)"=w242, "name (\"\")"="Setup" ("name (\"\")")) -> ("report out"=w240:refnum<class "NI_report.lvclass">, "error out"=w241:errorcluster)  [unwired: 11 in]
        n61 = Format Date/Time String(time format string (%c)="Bose Report_%H.%M.%S.xlsx") -> (date/time string=w250:string)  [unwired: 2 in]
        n62 = Build Path(base path=w246, name or relative path=w250) -> (appended path=w249:path)
        n63 = call-dynamic "Save Report to File.vi"("report in"=w240, "report file path"=w249, "error in (no error)"=w241) -> ("report out"=w254:refnum<class "NI_report.lvclass">, "error out"=w253:errorcluster)  [unwired: 2 in, 9 out]
        n64 = call-dynamic "Dispose Report.vi"("report in"=w254, "save changes? (F)"=w247, "error in (no error)"=w253, "close report? (T)"=w247) -> ("error out"=w252:errorcluster)  [unwired: 1 in, 10 out]
      }
    }
  }
  "error out" <- w6
